vi "SCCT Initialize.vi"(9 "API-Key":string="sensorNetwork", 10 "publisherPort":u16=8088, 11 "description":string="LabView") -> (0 "error out":errorcluster, 3 "publisher out":refnum<class "Publisher.lvclass">)   [LabVIEW 2011]
uses:
  <vilib>/TOOLS FOR SMART MINDS/SCCT/Publisher/Publisher.lvclass
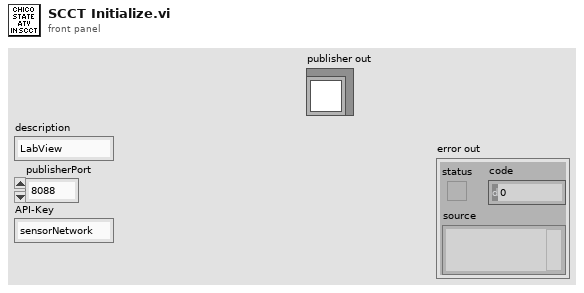
[diagram p1: front panel]
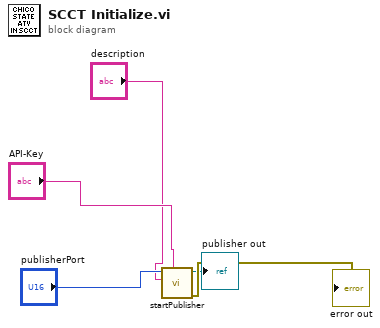
[diagram p0: block diagram]
diagram:
  n1 = call <vilib>:"startPublisher.vi"("API-Key"="API-Key", "description"="description", "port"="publisherPort") -> ("error out"=→"error out":errorcluster, "publisher out"=→"publisher out":refnum<class "Publisher.lvclass">)  [unwired: 7 in]
